vi "Condition disabled to none.vi"(8 "error in (no error)":errorcluster, 11 "Motor in":refnum<class "Motor.lvclass">) -> (0 "error out":errorcluster, 3 "Motor out":refnum<class "Motor.lvclass">)   [LabVIEW 2018, in "Motor.lvclass"]
uses:
  Motor.lvclass
  Motor.lvclass/Motor.ctl
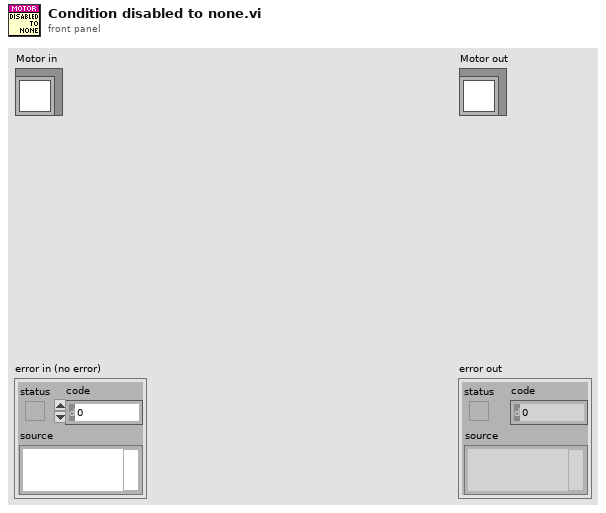
[diagram p1: front panel]
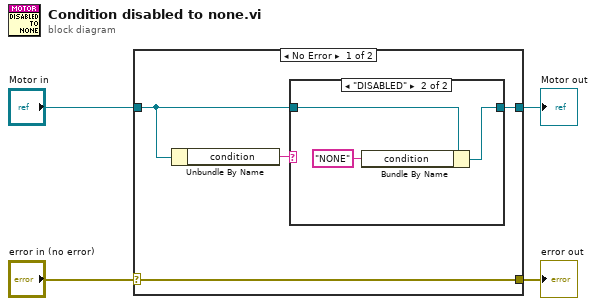
[diagram p0: block diagram]
diagram:
  n1 = case shown="No Error" "error in (no error)" {
    selector: "error in (no error)" -> [w8 w13]
    tunnel: [w8 w13] -> w3
    tunnel: [w6 w14] -> w1
    tunnel: "Motor in" -> [w7 w14]
    frame No Error {
      n2 = Unbundle By Name(w7) -> ("condition"=w5:string)
      n3 = case shown="\"DISABLED\"" w5 {
        tunnel: w7 -> [w9 w12]
        tunnel: [w9 w11] -> w6
        frame "NONE", Default {
        }
        frame "DISABLED" {
          n4 = Bundle By Name(cluster=w12, "condition"="NONE") -> (w11:refnum<class "Motor.lvclass">)
        }
      }
    }
    frame Error {
    }
  }
  "error out" <- w3
  "Motor out" <- w1
